vi "VNA.Configuration Window.vi"(8 "error in (no error)":errorcluster, 10 "Ex Configuration":T1, 11 "VNA":refnum<class "VNA.lvclass">) -> (0 "error out":errorcluster, 2 "output cluster":T1, 3 "VNA out":refnum<class "VNA.lvclass">)   [LabVIEW 2016, in "VNA.lvclass"]
uses:
  VNA.lvclass
  Typedefs/VNA.Configuration--Cluster.ctl
panel:
  in  "Example Setting 3":string
  in  "Example Setting 2":dbl
  in  "Example Setting 1":dbl
  in  "Cancel":bool
  in  "OK":bool
  # "confirm or make changes:"
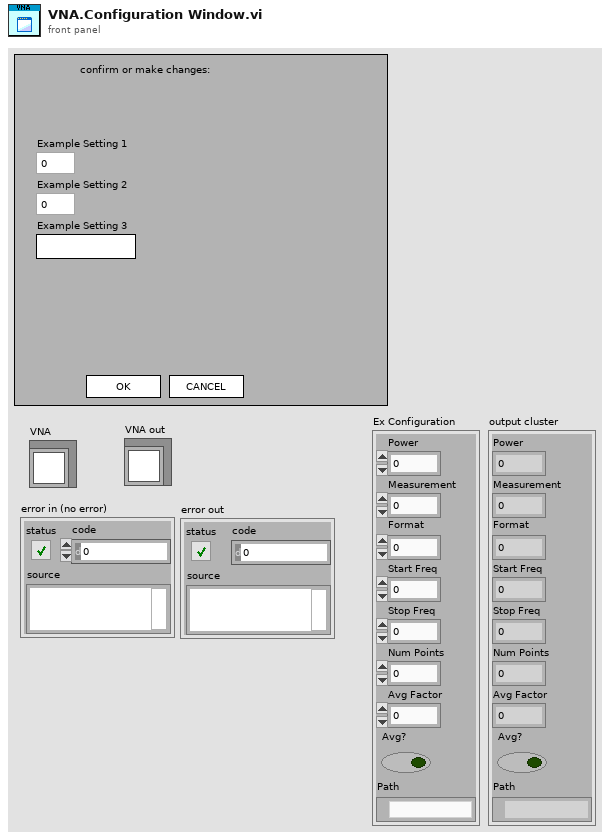
[diagram p1: front panel]
types:
  T1 = typedef "VNA.lvclass/VNA.Configuration--Cluster.ctl" = cluster{"Power":dbl, "Measurement":dbl, "Format":dbl, "Start Freq":dbl, "Stop Freq":dbl, "Num Points":dbl, "Avg Factor":dbl, "Avg?":bool, "Path":path}
  T2 = enum32{"Invalid", "Standard", "Closed", "Hidden", "Minimized", "Maximized"}
  T3 = enum32{"invalid app kind", "Development System", "Run Time System", "Student Edition", "Embedded LabVIEW", "Evaluation", "Custom"}
  T4 = cluster{"Core":cluster{"Current VI Reference":refnum<vi>, "Close Panel on Exit?":bool}, "Ex Configuration":T1}
  T5 = cluster{"Current VI Reference":refnum<vi>, "Close Panel on Exit?":bool}
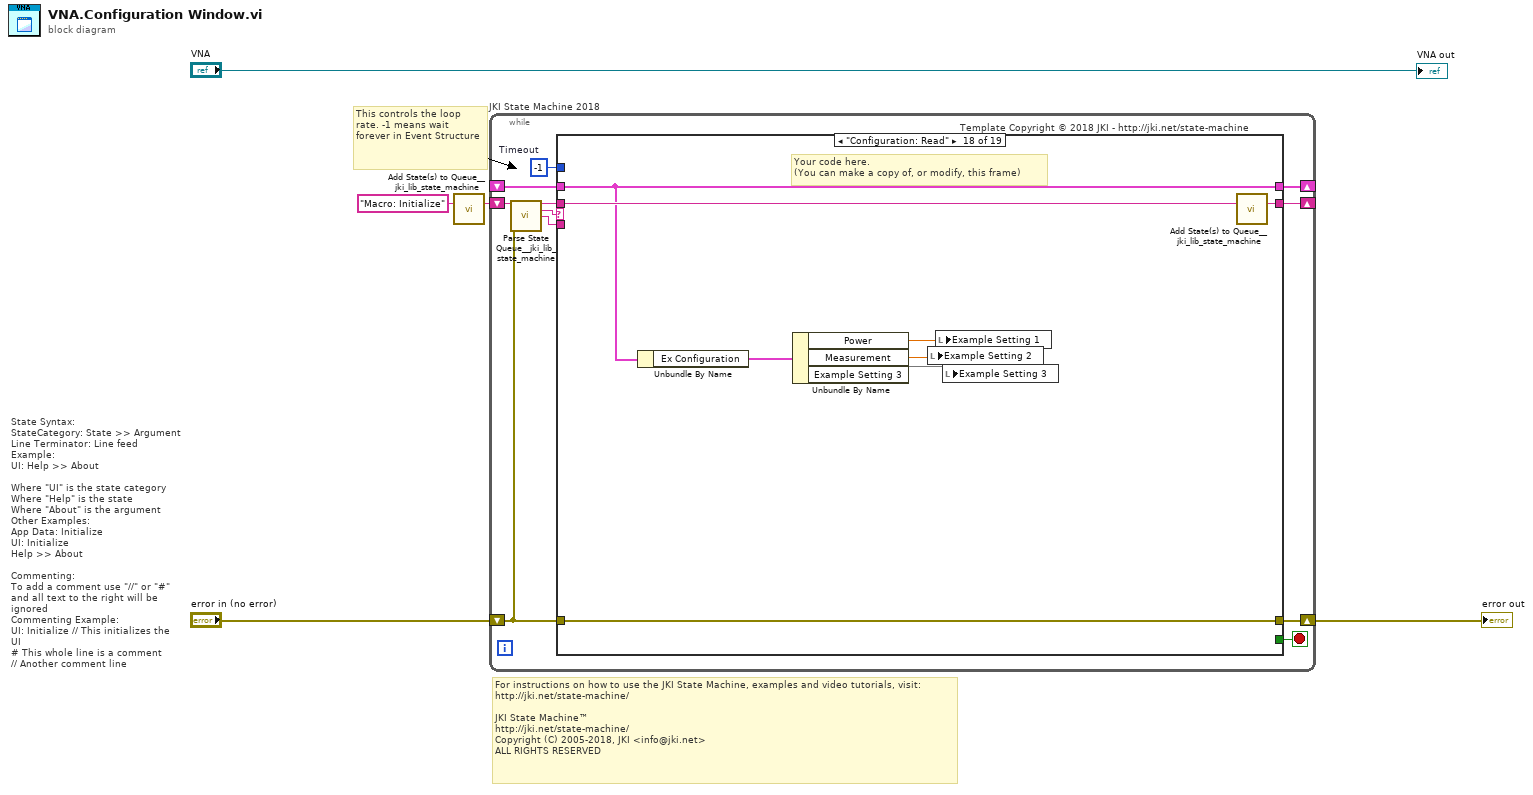
[diagram p0: block diagram]
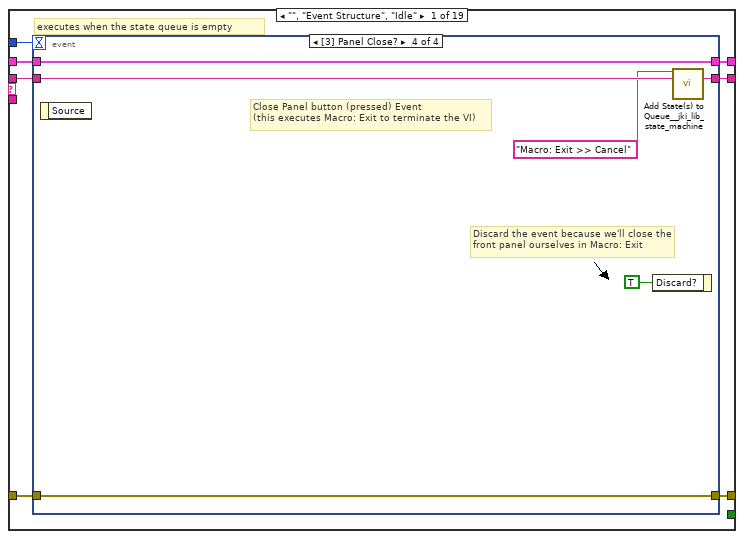
[diagram p2: hidden frame]
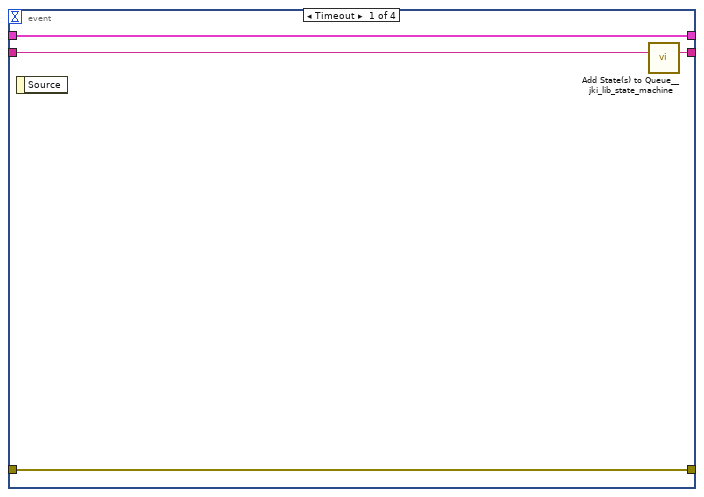
[diagram p3: hidden frame]
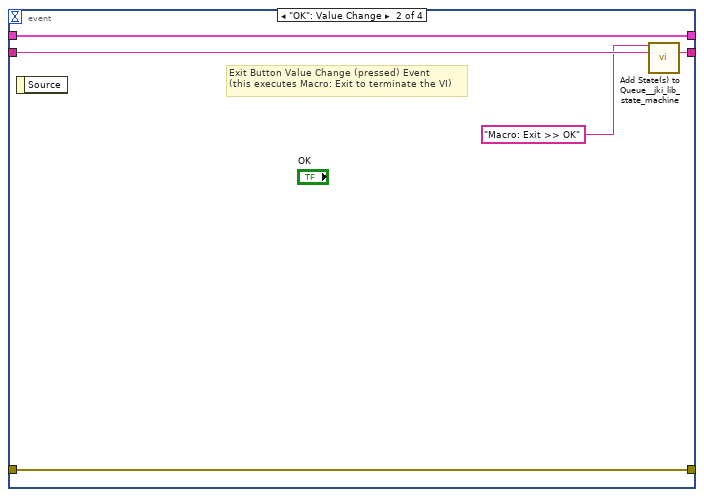
[diagram p4: hidden frame]
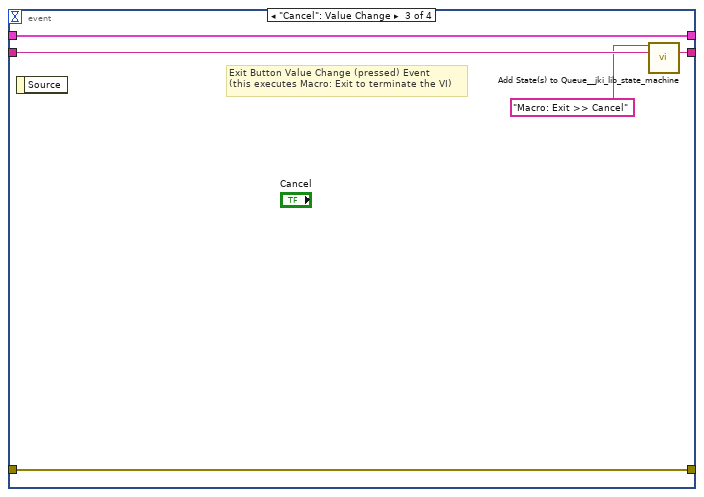
[diagram p5: hidden frame]
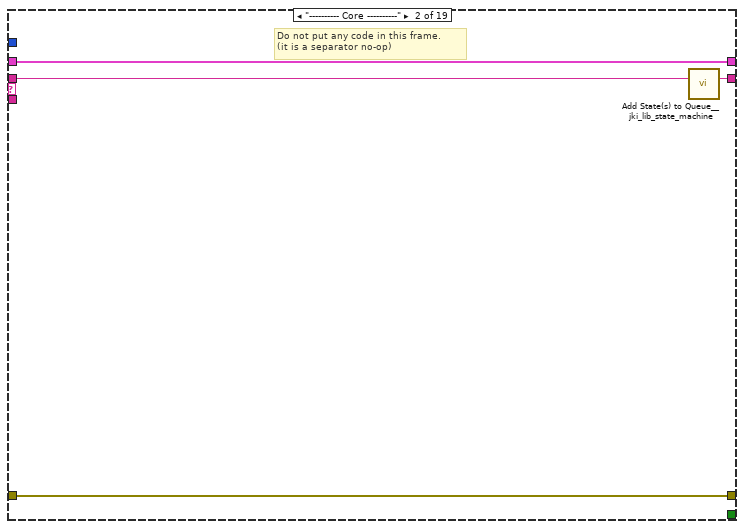
[diagram p6: hidden frame]
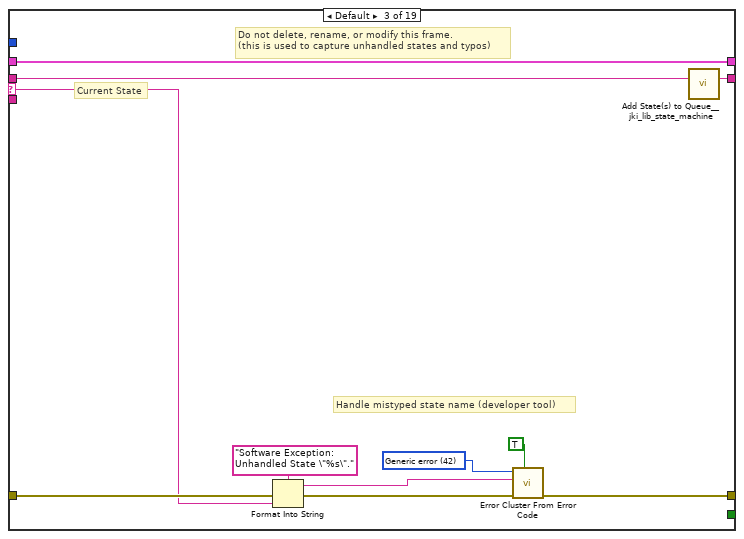
[diagram p7: hidden frame]
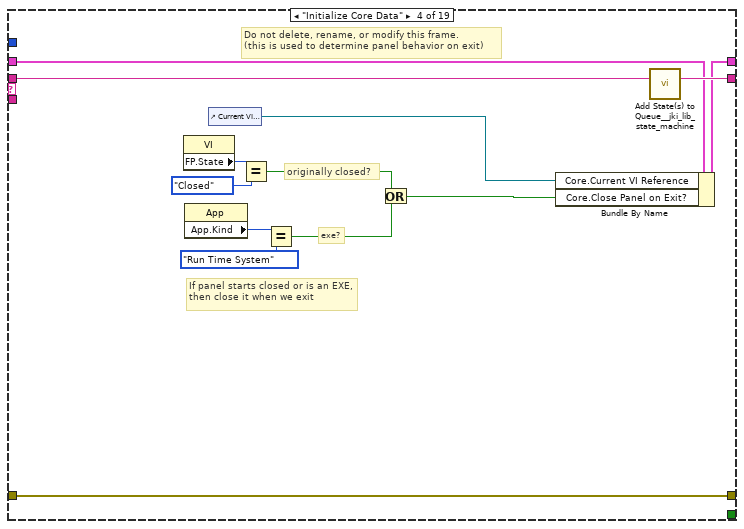
[diagram p8: hidden frame]
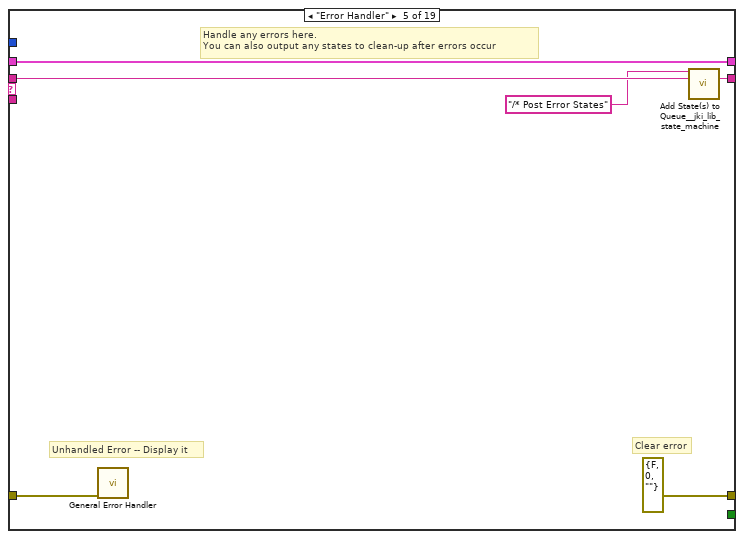
[diagram p9: hidden frame]
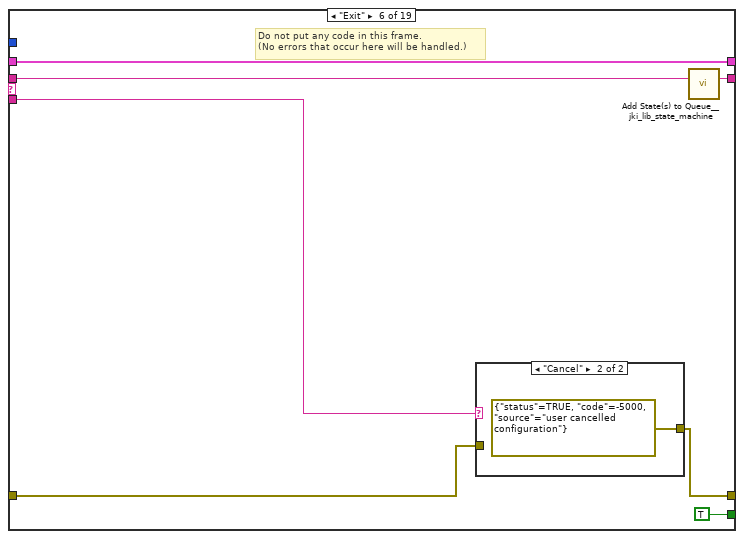
[diagram p10: hidden frame]
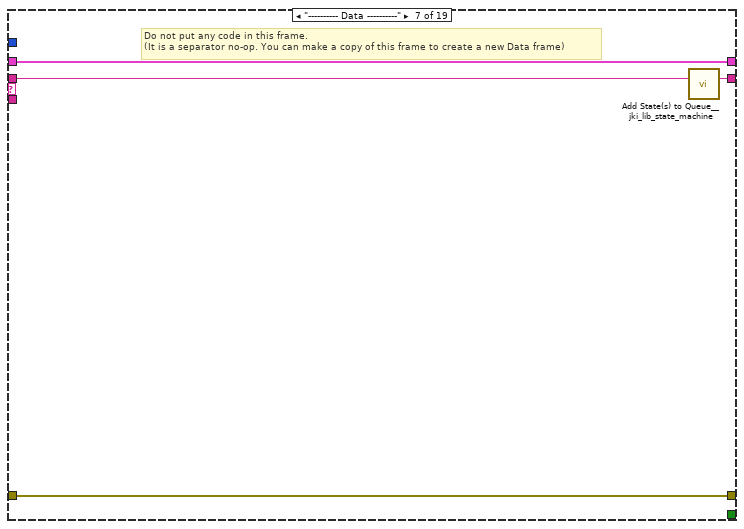
[diagram p12: hidden frame]
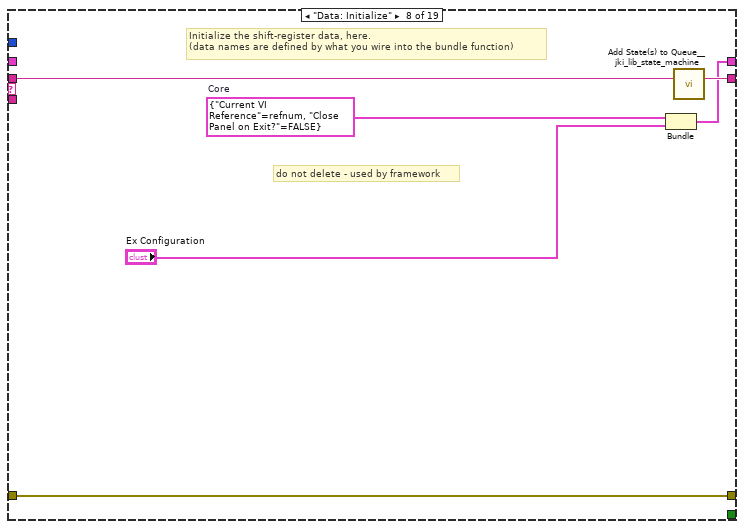
[diagram p13: hidden frame]
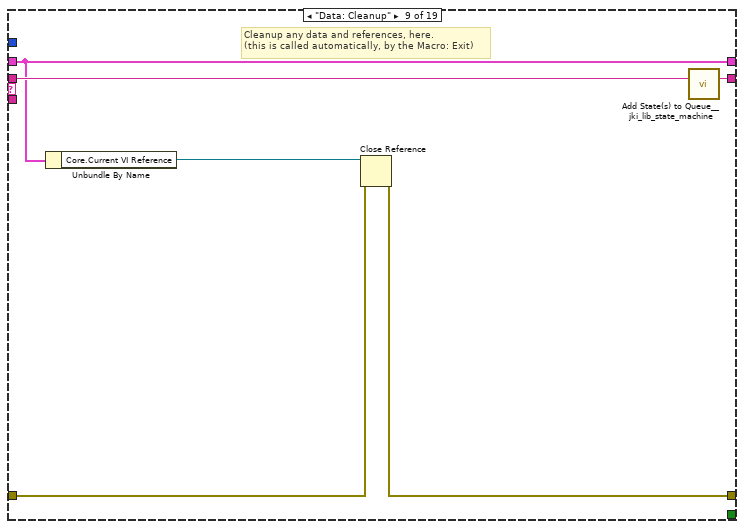
[diagram p14: hidden frame]
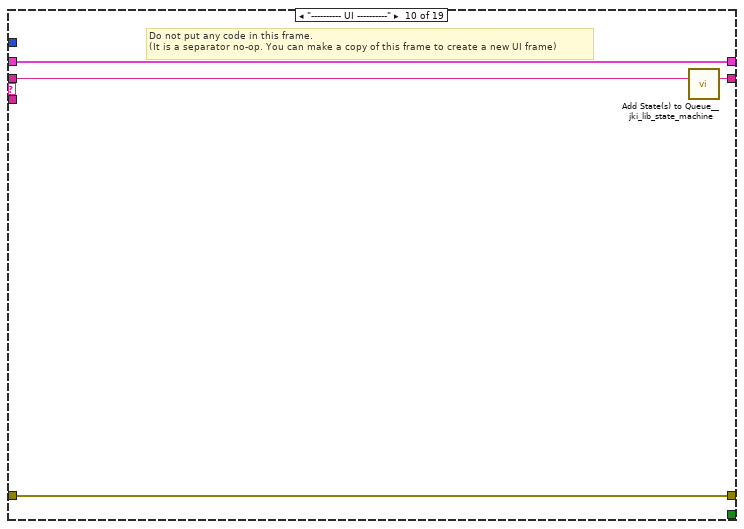
[diagram p15: hidden frame]
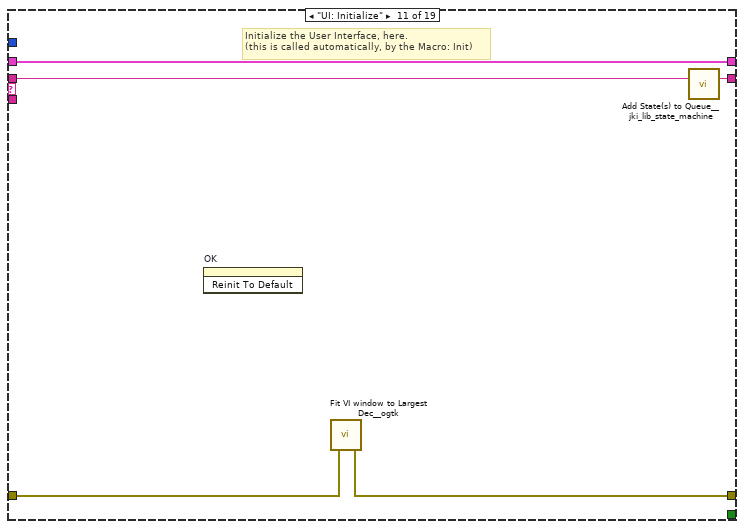
[diagram p16: hidden frame]
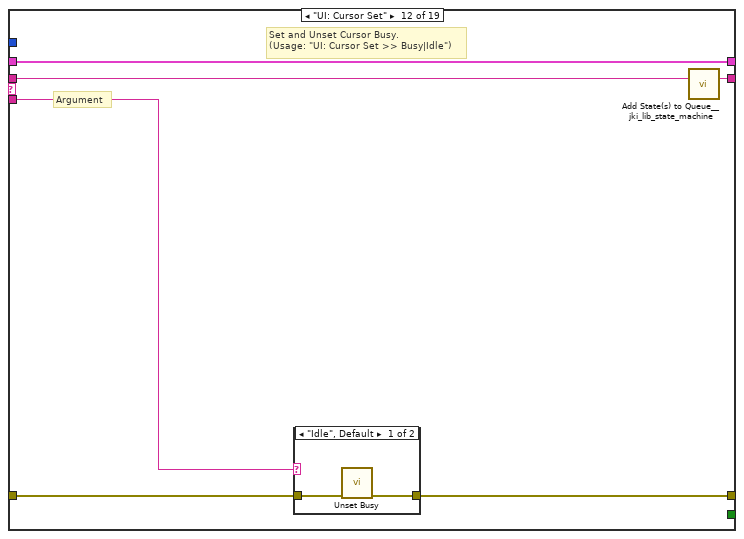
[diagram p17: hidden frame]
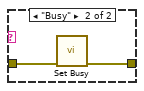
[diagram p18: hidden frame]
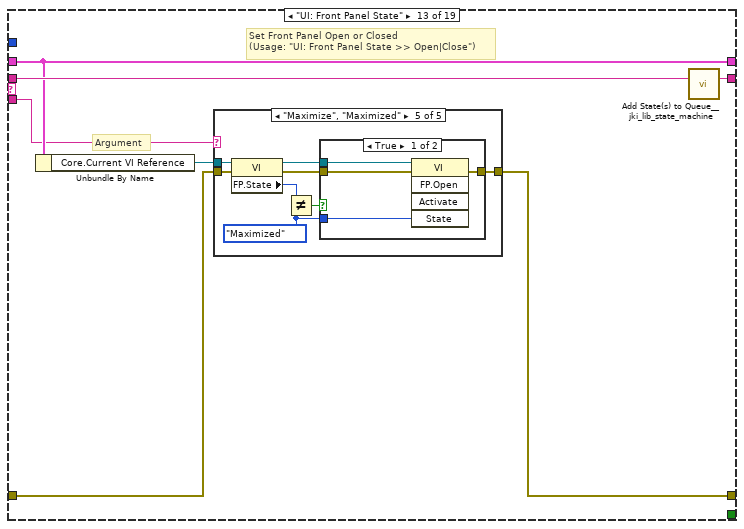
[diagram p19: hidden frame]
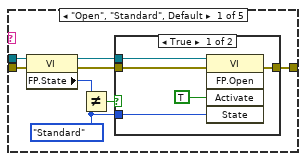
[diagram p20: hidden frame]
diagram:
  # "For instructions on how to use the JKI State Machine, examples and video tutorials, visit:\nhttp://jki.net/state-machine/\n\nJKI State Machine™\nhttp://jki.net/state-machine/\nCopyright (C) 2005-2018, JKI <info@jki.net>\nALL RIGHTS RESERVED"
  # "State Syntax:\nStateCategory: State >> Argument\nLine Terminator: Line feed\nExample:\nUI: Help >> About\n\nWhere \"UI\" is the state category\nWhere \"Help\" is the state\nWhere \"About\" is the argument\nOther Examples:\nApp Data: Initialize\nUI: Initialize\nHelp >> About\n\nCommenting:\nTo add a comment use \"//\" or \"#\" and all text to the right will be ignored\nCommenting Example:\nUI: Initialize // This initializes the UI\n# This whole line is a comment\n// Another comment line"
  # "This controls the loop rate. -1 means wait forever in Event Structure"
  n1 = call <vilib>:"Add State(s) to Queue__jki_lib_state_machine.vi"("State(s) in (\"\")"="Macro: Initialize") -> ("States Out"=w5:string)  [unwired: 14 in]
  n2 = while "JKI State Machine 2018" {
    shift-right: [w9] -> _
    shift-left: _ -> [w8]
    shift-right: [w12] -> w3
    shift-left: "error in (no error)" -> [w6]
    shift-right: [w11] -> _
    shift-left: w5 -> [w13]
    stop <- w10 stop-if-true
    w7 = -1  # Timeout
    # "Template Copyright © 2018 JKI - http://jki.net/state-machine"
    n3 = call <vilib>:"Parse State Queue__jki_lib_state_machine.vi"("State Queue"=w13, "Error In (no error)"=w6) -> ("Remaining States"=w15:string, "Current State"=w16:string, "Arguments"=w14:string)  [unwired: 11 in]
    n4 = case shown="\"Configuration: Read\"" w16 {
      selector: w16 -> [_ _ w48 _ _ _ _ _ _ _ _ _ _ _ _ _ _ _ _]
      tunnel: w15 -> [w23 w47 w52 w71 w77 w84 w90 w96 w102 w106 w111 w117 w128 w197 w202 w217 w221 w229 w237]
      tunnel: w14 -> [_ _ _ _ _ w80 _ _ _ _ _ w112 w122 _ _ w206 _ _ _]
      tunnel: w8 -> [w21 w44 w50 w64 w74 w82 w87 _ w97 w103 w109 w115 w124 w194 w199 w214 w218 w223 w233]
      tunnel: [w20 w45 w54 w68 errorcluster {"status"=FALSE, "code"=0, "source"=""} ("error out") w78 w88 w92 w98 w104 w107 w113 w125 w195 w200 w215 w219 w227 w235] -> w12
      tunnel: w6 -> [w19 w45 w53 w68 w73 w79 w88 w92 w99 w104 w108 w114 w126 w195 w200 w215 w219 w227 w235]
      tunnel: [w22 w46 w51 w70 w76 w83 w89 w95 w101 w105 w110 w116 w127 w196 w201 w216 w220 w228 w236] -> w11
      tunnel: [_ _ _ _ _ TRUE _ _ _ _ _ _ _ _ _ _ _ _ _] -> w10
      tunnel: [w18 w44 w50 w69 w74 w82 w87 w94 w97 w103 w109 w115 w124 w194 w199 w214 w218 w223 w233] -> w9
      tunnel: w7 -> [w17 _ _ _ _ _ _ _ _ _ _ _ _ _ _ _ _ _ _]
      frame "", "Event Structure", "Idle" {
        # "executes when the state queue is empty"
        n5 = event shown="[3] Panel Close?" {
          selector: _ -> [_ _ _ _]
          dyn-events: _ -> [_ _ _ _]
          timeout: w17 -> [_ _ _ _]
          tunnel: w23 -> [w27 w32 w37 w43]
          tunnel: [w26 w31 w36 w42] -> w22
          tunnel: w21 -> [w24 w29 w34 w40]
          tunnel: [w25 w30 w35 w41] -> w20
          tunnel: w19 -> [w25 w30 w35 w41]
          tunnel: [w24 w29 w34 w40] -> w18
          event Timeout {
            n6 = event-data() -> ()  [unwired: 1 in, 1 out]
            n7 = call <vilib>:"Add State(s) to Queue__jki_lib_state_machine.vi"("State(s) in (\"\")"=w27) -> ("States Out"=w26:string)  [unwired: 14 in]
          }
          event "OK": Value Change {
            # "Exit Button Value Change (pressed) Event\n(this executes Macro: Exit to terminate the VI)"
            n8 = event-data() -> ()  [unwired: 1 in, 1 out]
            n9 = call <vilib>:"Add State(s) to Queue__jki_lib_state_machine.vi"("State(s) in Front (\"\")"="Macro: Exit >> OK", "State(s) in (\"\")"=w32) -> ("States Out"=w31:string)  [unwired: 13 in]
          }
          event "Cancel": Value Change {
            # "Exit Button Value Change (pressed) Event\n(this executes Macro: Exit to terminate the VI)"
            n10 = event-data() -> ()  [unwired: 1 in, 1 out]
            n11 = call <vilib>:"Add State(s) to Queue__jki_lib_state_machine.vi"("State(s) in Front (\"\")"="Macro: Exit >> Cancel", "State(s) in (\"\")"=w37) -> ("States Out"=w36:string)  [unwired: 13 in]
          }
          event Panel Close? {
            # "Discard the event because we'll close the front panel ourselves in Macro: Exit"
            # "Close Panel button (pressed) Event\n(this executes Macro: Exit to terminate the VI)"
            n12 = event-data() -> ()  [unwired: 1 in, 1 out]
            n13 = event-data("Discard?"=TRUE) -> ()  [unwired: 1 in, 1 out]
            n14 = call <vilib>:"Add State(s) to Queue__jki_lib_state_machine.vi"("State(s) in Front (\"\")"="Macro: Exit >> Cancel", "State(s) in (\"\")"=w43) -> ("States Out"=w42:string)  [unwired: 13 in]
          }
        }
      }
      frame "---------- Core ----------" {
        # "Do not put any code in this frame.\n(it is a separator no-op)"
        n15 = call <vilib>:"Add State(s) to Queue__jki_lib_state_machine.vi"("State(s) in (\"\")"=w47) -> ("States Out"=w46:string)  [unwired: 14 in]
      }
      frame Default {
        w57 = 42 items=["No error", "Argument error", "Memory is full", "Out of zone", "End of file", "File already open", "Generic file I/O error", "File not found", "File permission error", "Disk is full", "Duplicate path", "Too many files open", "System feature not enabled", "Resource file not found", "Cannot add resource", "Resource not found", "Image not found", "Image memory error", "Pen does not exist", "Config type invalid", "Config token not found", "Config parse error", "Config memory error", "Bad external code format", "Bad external code offset", "External code not present", "Null window", "Destroy window error", "Null menu", "Print aborted", "Bad print record", "Print driver error", "Windows error during printing", "Memory error during printing", "Print dialog error", "Generic print error", "Invalid device refnum", "Device not found", "Device parameter error", "Device unit error", "Cannot open device", "Device call aborted", "Generic error", "Cancelled by user", "Object ID too low", "Object ID too high", "Object not in heap", "Unknown heap", "Unknown object (invalid DefProc)", "Unknown object (DefProc not in table)", "Message out of range", "Invalid (null) method", "Unknown message", "Manager call not supported", "Bad address", "Network operation in progress", "Network operation timed out", "Connection is busy", "Network attribute not supported", "Network error", "Address in use", "System out of memory", "Connection aborted", "Connection refused", "Not connected", "Already connected", "Connection closed", "Initialization error (interapplication manager)", "Bad occurrence", "Wait on unbound occurrence handler", "Occurrence queue overflow", "Datalog type conflict", "Unused", "Unrecognized type (interapplication manager)", "Memory corrupt", "Failed to make temporary DLL", "Old CIN version", "Drag socket not found", "Failed to load drop-object", "Failed to register OLE object", "Failed to release OLE object", "Format specifier type mismatch", "Unknown format specifier", "Too few format specifiers", "Too many format specifiers", "Scan failed", "Newer CIN version", "Error converting to variant", "Runtime menu error", "Password tampered", "Variant attribute not found", "Incompatible variant data type", "Event data is not available", "Event Store is not present", "Occurrence is not found", "Event Queue is not created", "Event info is not available", "Refnum passed is NULL", "Error retrieving Class GUID", "Error retrieving CoClass GUID", "Error retrieving TypeLib GUID.", "Bad built application magic bytes.", "Specific driver is different from the specific driver associated with the Logical Name.", "There is no session opened to the class driver.", "Max Error", "MAX - Error with config objects", "MAX - Error loading configuration", "MAX - Group not supported"]
        # "Current State"
        # "Do not delete, rename, or modify this frame.\n(this is used to capture unhandled states and typos)"
        # "Handle mistyped state name (developer tool)"
        n16 = Format Into String(format string="Software Exception: Unhandled State \"%s\"." ("message"), error in=w53, w48) -> (resulting string=w56:string, error out=w55:errorcluster)  [unwired: 1 in]
        n17 = call <vilib>:"Error Cluster From Error Code.vi"("show call chain? (False)"=TRUE, "error in (no error)"=w55, "error message (\"\")"=w56, "error code (0)"=w57) -> ("error out"=w54:errorcluster)  [unwired: 5 in]
        n18 = call <vilib>:"Add State(s) to Queue__jki_lib_state_machine.vi"("State(s) in (\"\")"=w52) -> ("States Out"=w51:string)  [unwired: 14 in]
      }
      frame "Initialize Core Data" {
        # "Do not delete, rename, or modify this frame.\n(this is used to determine panel behavior on exit)"
        # "originally closed?"
        # "exe?"
        # "If panel starts closed or is an EXE, then close it when we exit"
        n19 = property class="VI"() -> ("FP.State"=w61:T2)  [unwired: 2 in, 2 out]
        n20 = property class="App"() -> ("App.Kind"=w67:T3)  [unwired: 2 in, 2 out]
        n21 = control-ref of="Current VI Reference"() -> (w62:refnum<vi>)
        n22 = Equal?(x=w61, y=T2."Closed" ("Front Panel Window:State")) -> (x = y?=w59:bool)
        n23 = Equal?(x=w67, y=T3."Run Time System" ("Application:Kind")) -> (x = y?=w65:bool)
        n24 = Or(x=w59, y=w65) -> (x .or. y?=w63:bool)
        n25 = Bundle By Name(cluster=w64, "Core.Current VI Reference"=w62, "Core.Close Panel on Exit?"=w63) -> (w69:T4)
        n26 = call <vilib>:"Add State(s) to Queue__jki_lib_state_machine.vi"("State(s) in (\"\")"=w71) -> ("States Out"=w70:string)  [unwired: 14 in]
      }
      frame "Error Handler" {
        # "Unhandled Error -- Display it"
        # "Handle any errors here.\nYou can also output any states to clean-up after errors occur"
        # "Clear error"
        n27 = call <vilib>:"General Error Handler.vi"("error in (no error)"=w73) -> ()  [unwired: 10 in, 5 out]
        n28 = call <vilib>:"Add State(s) to Queue__jki_lib_state_machine.vi"("State(s) in Front (\"\")"="/* Post Error States", "State(s) in (\"\")"=w77) -> ("States Out"=w76:string)  [unwired: 13 in]
      }
      frame "Exit" {
        # "Do not put any code in this frame.\n(No errors that occur here will be handled.)"
        n29 = case shown="\"Cancel\"" w80 {
          tunnel: w79 -> [w85 _]
          tunnel: [w85 errorcluster {"status"=TRUE, "code"=-5000, "source"="user cancelled configuration"} ("error in (no error)")] -> w78
          frame "OK", Default {
          }
          frame "Cancel" {
          }
        }
        n30 = call <vilib>:"Add State(s) to Queue__jki_lib_state_machine.vi"("State(s) in (\"\")"=w84) -> ("States Out"=w83:string)  [unwired: 14 in]
      }
      frame "---------- Data ----------" {
        # "Do not put any code in this frame.\n(It is a separator no-op. You can make a copy of this frame to create a new Data frame)"
        n31 = call <vilib>:"Add State(s) to Queue__jki_lib_state_machine.vi"("State(s) in (\"\")"=w90) -> ("States Out"=w89:string)  [unwired: 14 in]
      }
      frame "Data: Initialize" {
        w93 = T5 {"Current VI Reference"=refnum, "Close Panel on Exit?"=FALSE}  # Core
        # "do not delete - used by framework"
        # "Initialize the shift-register data, here.\n(data names are defined by what you wire into the bundle function)"
        n32 = Bundle("Core"=w93, "Ex Configuration"="Ex Configuration") -> (w94:T4)  [unwired: 1 in]
        n33 = call <vilib>:"Add State(s) to Queue__jki_lib_state_machine.vi"("State(s) in (\"\")"=w96) -> ("States Out"=w95:string)  [unwired: 14 in]
      }
      frame "Data: Cleanup" {
        # "Cleanup any data and references, here.\n(this is called automatically, by the Macro: Exit)"
        n34 = Unbundle By Name(w97) -> ("Core.Current VI Reference"=w100:refnum<vi>)
        n35 = Close Reference(reference=w100, error in (no error)=w99) -> (error out=w98:errorcluster)
        n36 = call <vilib>:"Add State(s) to Queue__jki_lib_state_machine.vi"("State(s) in (\"\")"=w102) -> ("States Out"=w101:string)  [unwired: 14 in]
      }
      frame "---------- UI ----------" {
        # "Do not put any code in this frame.\n(It is a separator no-op. You can make a copy of this frame to create a new UI frame)"
        n37 = call <vilib>:"Add State(s) to Queue__jki_lib_state_machine.vi"("State(s) in (\"\")"=w106) -> ("States Out"=w105:string)  [unwired: 14 in]
      }
      frame "UI: Initialize" {
        # "Initialize the User Interface, here.\n(this is called automatically, by the Macro: Init)"
        n38 = invoke on="OK" class="Bool" method="Reinit To Default"() -> ()  [unwired: 3 in, 3 out]
        n39 = call <userlib>:"Fit VI window to Largest Dec__ogtk.vi"("error in (no error)"=w108) -> ("error out"=w107:errorcluster)  [unwired: 5 in, 1 out]
        n40 = call <vilib>:"Add State(s) to Queue__jki_lib_state_machine.vi"("State(s) in (\"\")"=w111) -> ("States Out"=w110:string)  [unwired: 14 in]
      }
      frame "UI: Cursor Set" {
        # "Argument"
        # "Set and Unset Cursor Busy.\n(Usage: \"UI: Cursor Set >> Busy|Idle\")"
        n41 = case shown="\"Idle\", Default" w112 {
          tunnel: w114 -> [w119 w121]
          tunnel: [w118 w120] -> w113
          frame "Idle", Default {
            n42 = call <vilib>:"Unset Busy.vi"("error in (no error)"=w119) -> ("error out"=w118:errorcluster)  [unwired: 10 in]
          }
          frame "Busy" {
            n43 = call <vilib>:"Set Busy.vi"("error in (no error)"=w121) -> ("error out"=w120:errorcluster)  [unwired: 9 in, 1 out]
          }
        }
        n44 = call <vilib>:"Add State(s) to Queue__jki_lib_state_machine.vi"("State(s) in (\"\")"=w117) -> ("States Out"=w116:string)  [unwired: 14 in]
      }
      frame "UI: Front Panel State" {
        # "Argument"
        # "Set Front Panel Open or Closed\n(Usage: \"UI: Front Panel State >> Open|Close\")"
        n45 = Unbundle By Name(w124) -> ("Core.Current VI Reference"=w123:refnum<vi>)
        n46 = case shown="\"Maximize\", \"Maximized\"" w122 {
          tunnel: w126 -> [w134 w149 w160 w173 w186]
          tunnel: [w136 w150 w162 w175 w188] -> w125
          tunnel: w123 -> [w135 w147 w161 w174 w187]
          frame "Open", "Standard", Default {
            w129 = T2."Standard" ("State")
            n47 = property class="VI"(reference=w135, error in=w134) -> (reference out=w132:refnum<vi>, error out=w133:errorcluster, "FP.State"=w131:T2)
            n48 = Not Equal?(x=w131, y=w129) -> (x != y?=w130:bool)
            n49 = case shown="True" w130 {
              tunnel: [w140 w142] -> w136
              tunnel: w133 -> [w139 w142]
              tunnel: w132 -> [w138 _]
              tunnel: w129 -> [w137 _]
              frame True {
                n50 = invoke class="VI" method="FP.Open"(reference=w138, error in=w139, "Activate"=TRUE, "State"=w137) -> (error out=w140:errorcluster)  [unwired: 1 in, 4 out]
              }
              frame False {
              }
            }
          }
          frame "Close", "Closed" {
            n51 = property class="VI"(reference=w147, error in=w149) -> (reference out=w146:refnum<vi>, error out=w148:errorcluster, "FP.State"=w144:T2)
            n52 = Not Equal?(x=w144, y=T2."Closed" ("Front Panel Window:State")) -> (x != y?=w143:bool)
            n53 = case shown="True" w143 {
              tunnel: [w151 w154] -> w150
              tunnel: w148 -> [w151 w153]
              tunnel: w146 -> [_ w152]
              frame False {
              }
              frame True {
                n54 = invoke class="VI" method="FP.Close"(reference=w152, error in=w153) -> (error out=w154:errorcluster)  [unwired: 1 in, 2 out]
              }
            }
          }
          frame "Hidden", "Hide" {
            w155 = T2."Hidden" ("State")
            n55 = property class="VI"(reference=w161, error in=w160) -> (reference out=w158:refnum<vi>, error out=w159:errorcluster, "FP.State"=w157:T2)
            n56 = Not Equal?(x=w157, y=w155) -> (x != y?=w156:bool)
            n57 = case shown="True" w156 {
              tunnel: [w166 w167] -> w162
              tunnel: w159 -> [w165 w167]
              tunnel: w158 -> [w164 _]
              tunnel: w155 -> [w163 _]
              frame True {
                n58 = invoke class="VI" method="FP.Open"(reference=w164, error in=w165, "State"=w163) -> (error out=w166:errorcluster)  [unwired: 2 in, 4 out]
              }
              frame False {
              }
            }
          }
          frame "Minimize", "Minimized" {
            w168 = T2."Minimized" ("State")
            n59 = property class="VI"(reference=w174, error in=w173) -> (reference out=w171:refnum<vi>, error out=w172:errorcluster, "FP.State"=w170:T2)
            n60 = Not Equal?(x=w170, y=w168) -> (x != y?=w169:bool)
            n61 = case shown="True" w169 {
              tunnel: [w179 w180] -> w175
              tunnel: w172 -> [w178 w180]
              tunnel: w171 -> [w177 _]
              tunnel: w168 -> [w176 _]
              frame True {
                n62 = invoke class="VI" method="FP.Open"(reference=w177, error in=w178, "State"=w176) -> (error out=w179:errorcluster)  [unwired: 2 in, 4 out]
              }
              frame False {
              }
            }
          }
          frame "Maximize", "Maximized" {
            w181 = T2."Maximized" ("State")
            n63 = property class="VI"(reference=w187, error in=w186) -> (reference out=w184:refnum<vi>, error out=w185:errorcluster, "FP.State"=w183:T2)
            n64 = Not Equal?(x=w183, y=w181) -> (x != y?=w182:bool)
            n65 = case shown="True" w182 {
              tunnel: [w192 w193] -> w188
              tunnel: w185 -> [w191 w193]
              tunnel: w184 -> [w190 _]
              tunnel: w181 -> [w189 _]
              frame True {
                n66 = invoke class="VI" method="FP.Open"(reference=w190, error in=w191, "State"=w189) -> (error out=w192:errorcluster)  [unwired: 2 in, 4 out]
              }
              frame False {
              }
            }
          }
        }
        n67 = call <vilib>:"Add State(s) to Queue__jki_lib_state_machine.vi"("State(s) in (\"\")"=w128) -> ("States Out"=w127:string)  [unwired: 14 in]
      }
      frame "---------- Macro ----------" {
        # "Do not put any code in this frame.\n(It is a separator no-op. You can make a copy of this frame to create a new Macro frame)"
        n68 = call <vilib>:"Add State(s) to Queue__jki_lib_state_machine.vi"("State(s) in (\"\")"=w197) -> ("States Out"=w196:string)  [unwired: 14 in]
      }
      frame "Macro: Initialize" {
        w198 = "Data: Initialize\nInitialize Core Data\nUI: Initialize\nUI: Front Panel State >> Open\nConfiguration: Read"  # Data: Initialize Initialize Core Data UI: Initialize UI: Front Panel State >> Open Configuration: Read
        # "Initialization Macro\n(This is called once, when the VI starts)"
        n69 = call <vilib>:"Add State(s) to Queue__jki_lib_state_machine.vi"("State(s) in Front (\"\")"=w198, "State(s) in (\"\")"=w202) -> ("States Out"=w201:string)  [unwired: 13 in]
      }
      frame "Macro: Exit" {
        # "Exit Macro\n(This is called once, when the VI exits)"
        n70 = Unbundle By Name(w214) -> ("Core.Close Panel on Exit?"=w213:bool)
        n71 = call <vilib>:"Build State String with Arguments__JKI_lib_State_Machine.vi"("Arguments (\"\")"=w206, "State"="Exit") -> ("State with Arguments"=w204:string)  [unwired: 4 in]
        n72 = Select(t="UI: Front Panel State >> Close", s=w213, f="") -> (s? t:f=w210:string)
        n73 = call <vilib>:"Add State(s) to Queue__jki_lib_state_machine.vi"("State(s) in Front (\"\")"="Data: Cleanup", "State(s) at Back (\"\")"=w204) -> ("States Out"=w203:string)  [unwired: 13 in]
        n74 = call <vilib>:"Add State(s) to Queue__jki_lib_state_machine.vi"("State(s) in Front (\"\")"="Configuration: Write", "State(s) in (\"\")"=w210, "State(s) at Back (\"\")"=w203) -> ("States Out"=w209:string)  [unwired: 12 in]
        n75 = call <vilib>:"Add State(s) to Queue__jki_lib_state_machine.vi"("State(s) in Front (\"\")"=w209, "State(s) in (\"\")"=w217) -> ("States Out"=w216:string)  [unwired: 13 in]
      }
      frame "---------- Configuration ----------" {
        # "Template Separator\n(You can make a copy of, or modify, this frame)"
        n76 = call <vilib>:"Add State(s) to Queue__jki_lib_state_machine.vi"("State(s) in (\"\")"=w221) -> ("States Out"=w220:string)  [unwired: 14 in]
      }
      frame "Configuration: Read" {
        # "Your code here.\n(You can make a copy of, or modify, this frame)"
        n77 = Unbundle By Name(w223) -> ("Ex Configuration"=w222:T1)
        n78 = Unbundle By Name(w222) -> ("Power"=w226:dbl, "Measurement"=w225:dbl, "Example Setting 3"=w224)
        n79 = local write "Example Setting 2"(w225) -> ()
        n80 = local write "Example Setting 1"(w226) -> ()
        n81 = local write "Example Setting 3"(w224) -> ()
        n82 = call <vilib>:"Add State(s) to Queue__jki_lib_state_machine.vi"("State(s) in (\"\")"=w229) -> ("States Out"=w228:string)  [unwired: 14 in]
      }
      frame "Configuration: Write" {
        n83 = local read "Example Setting 1"() -> (w234:dbl)
        n84 = local read "Example Setting 2"() -> (w231:dbl)
        n85 = Unbundle By Name(w233) -> ("Ex Configuration"=w232:T1)
        n86 = Bundle By Name(cluster=w232, "Power"=w234, "Measurement"=w231) -> (→"output cluster":T1)  [unwired: 1 in]
        n87 = call <vilib>:"Add State(s) to Queue__jki_lib_state_machine.vi"("State(s) in (\"\")"=w237) -> ("States Out"=w236:string)  [unwired: 14 in]
      }
    }
  }
  "error out" <- w3
  "VNA out" <- "VNA"
